vi "cwd.vi"   [LabVIEW 2015, in "TestLib.lvlib"]
uses:
  TestLib.lvlib
  CLI Class/CLI.lvclass
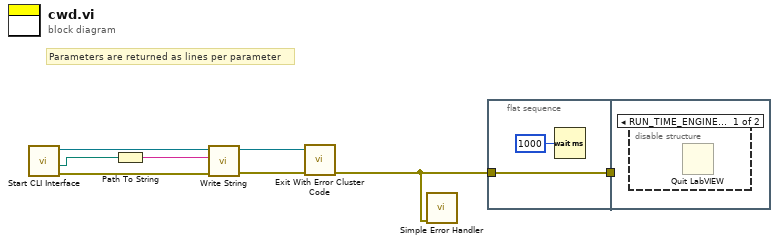
[diagram p0: block diagram]
diagram:
  # "Parameters are returned as lines per parameter"
  n1 = call "Start CLI Interface.vi"() -> ("error out"=w4:errorcluster, "Working Directory"=w2:path, "CLI out"=w5:refnum<class "CLI.lvclass">)  [unwired: 8 in, 1 out]
  n2 = Path To String(path=w2) -> (string=w1:string)
  n3 = call "Write String.vi"("error in (no error)"=w4, "Text to Write"=w1, "CLI in"=w5) -> ("error out"=w7:errorcluster, "CLI out"=w6:refnum<class "CLI.lvclass">)  [unwired: 7 in]
  n4 = call "Exit With Error Cluster Code.vi"("error in (no error)"=w7, "CLI in"=w6) -> ("error out"=w3:errorcluster)  [unwired: 9 in]
  n5 = call <vilib>:"Simple Error Handler.vi"("error in (no error)"=w3) -> ()  [unwired: 4 in, 5 out]
  n6 = flat-sequence {
    tunnel: w3 -> [w10]
    tunnel: [w10] -> w8
    tunnel: w8 -> [_]
    frame #0 {
      n7 = Wait (ms)(milliseconds to wait=u32 1000) -> ()  [unwired: 1 out]
    }
    frame #1 {
      n8 = disable-structure shown="RUN_TIME_ENGINE==True" {
        frame condition #0 {
          n9 = Quit LabVIEW() -> ()  [unwired: 1 in]
        }
        frame condition #1 (active) {
        }
      }
    }
  }
